vi "LHF.DB.Mongo.Collection.JSON.FindOneById.vi"(6 "Extract _id (T)":bool=TRUE, 7 "type":variant, 8 "error in (no error)":errorcluster, 9 "_id":string, 10 "Collection":string, 11 "LHF.DB.Mongo in":refnum<class "LHF.DB.Mongo.lvclass">) -> (0 "error out":errorcluster, 1 "_id":string, 2 "JSON Document":string, 3 "LHF.DB.Mongo out":refnum<class "LHF.DB.Mongo.lvclass">)   [LabVIEW 2013, in "LHF.DB.Mongo.lvclass"]
uses:
  LHF.DB.Mongo.lvclass
  C:/Users/Ricardo/Desktop/Projetos/LabVIEW-MongoDB/src/Driver/MongoDB.Bson.dll
  Driver/MongoDB.Bson.dll
  C:/Users/Ricardo/Desktop/Projetos/LabVIEW-MongoDB/src/Driver/MongoDB.Driver.dll
  Driver/MongoDB.Driver.dll
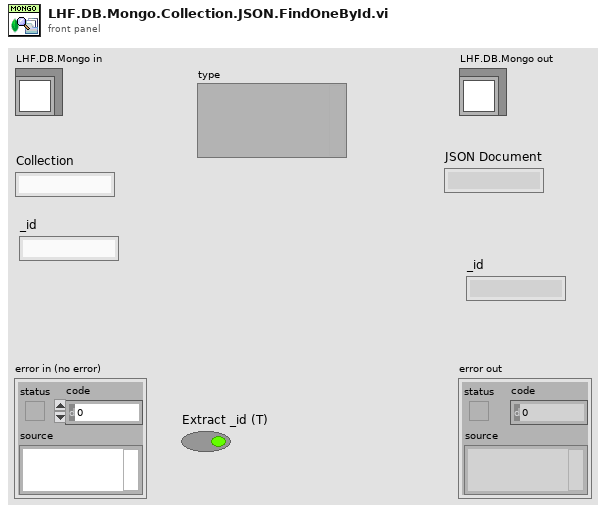
[diagram p1: front panel]
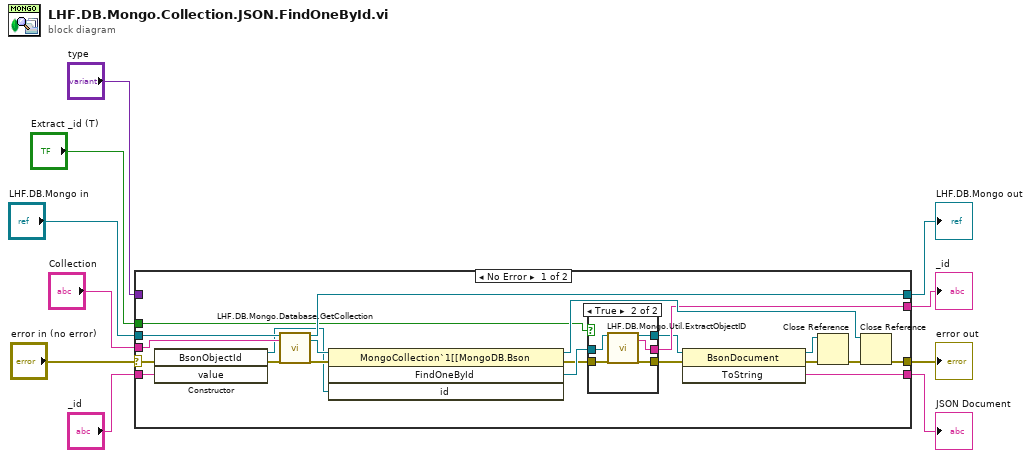
[diagram p0: block diagram]
diagram:
  n1 = case shown="No Error" "error in (no error)" {
    selector: "error in (no error)" -> [w19 w40]
    tunnel: [w27 w40] -> w1
    tunnel: [w30 w39] -> w8
    tunnel: "LHF.DB.Mongo in" -> [w29 w39]
    tunnel: "Collection" -> [w31 _]
    tunnel: [w22 _] -> w6
    tunnel: "_id" -> [w21 _]
    tunnel: "Extract _id (T)" -> [w17 _]
    tunnel: "type" -> [_ _]
    tunnel: [w11 _] -> w2
    frame No Error {
      n2 = constructor class="BsonObjectId"(error in=w19, "value"=w21) -> (reference out=w20:refnum<k24>, error out=w18:errorcluster)  [unwired: 2 in, 2 out]
      n3 = call "LHF.DB.Mongo.Database.GetCollection.vi"("LHF.DB.Mongo in"=w29, "collectionName"=w31, "error in (no error)"=w18) -> ("LHF.DB.Mongo in"=w30:refnum<class "LHF.DB.Mongo.lvclass">, "MongoCollection"=w26:refnum<k24>, "error out"=w25:errorcluster)  [unwired: 14 in]
      n4 = invoke class="MongoCollection`1[[MongoDB.Bson" method="FindOneById"(reference=w26, error in=w25, "id"=w20) -> (reference out=w28:refnum<k24>, error out=w16:errorcluster, "FindOneById"=w24:refnum<k24>)  [unwired: 1 in, 1 out]
      n5 = case shown="True" w17 {
        tunnel: [w33 w38] -> w13
        tunnel: [w32 w37] -> w15
        tunnel: w24 -> [w33 w36]
        tunnel: [_ w35] -> w22
        tunnel: w16 -> [w32 w34]
        frame False {
        }
        frame True {
          n6 = call "LHF.DB.Mongo.Util.ExtractObjectID.vi"("BsonDocument Refnum in"=w36, "error in (no error)"=w34) -> ("BsonDocument Refnum out"=w38:refnum<k24>, "_id"=w35:string, "error out"=w37:errorcluster)  [unwired: 15 in]
        }
      }
      n7 = invoke class="BsonDocument" method="ToString"(reference=w13, error in=w15) -> (reference out=w12:refnum<k24>, error out=w14:errorcluster, "ToString"=w11:string)  [unwired: 1 in]
      n8 = Close Reference(reference=w12, error in (no error)=w14) -> (error out=w23:errorcluster)
      n9 = Close Reference(reference=w28, error in (no error)=w23) -> (error out=w27:errorcluster)
    }
    frame Error {
    }
  }
  "error out" <- w1
  "LHF.DB.Mongo out" <- w8
  "JSON Document" <- w2
  "_id" <- w6
